vi "Set V1 (SubVI).vi"(11 "Voltage X":string) -> (3 "String":string)   [LabVIEW 2018]
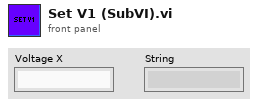
[diagram p1: front panel]
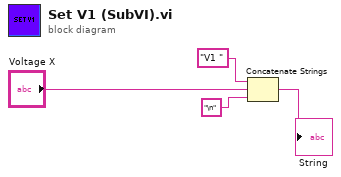
[diagram p0: block diagram]
diagram:
  n1 = Concatenate Strings("V1 ", "Voltage X", "\n") -> (→"String":string)
